vi "Test Save Animated GIF (Path).vi"(8 "error in (no error)":errorcluster) -> (0 "error out":errorcluster, 3 "Pass?":bool)   [LabVIEW 2020]
uses:
  G-Image/Image IO/Controls/Dither Type.ctl
  0f1b1910-5d7c-4507-bdef-12e0c9c3451f.vi
  G-Image/Image IO/Polymorphic VIs/Save Animated GIF Image (Path).vi
  G-Image/Image IO/Polymorphic VIs/Load Animated GIF Image (Path).vi
  G-Image/G-Image.lvlib
panel:
  out "Waveform Chart":cluster{dbl, dbl}(graph)={-0.06975647374412564, 0.4806308479691592}
  out "Array":cluster{string, "new picture":picture}[](array[cluster])
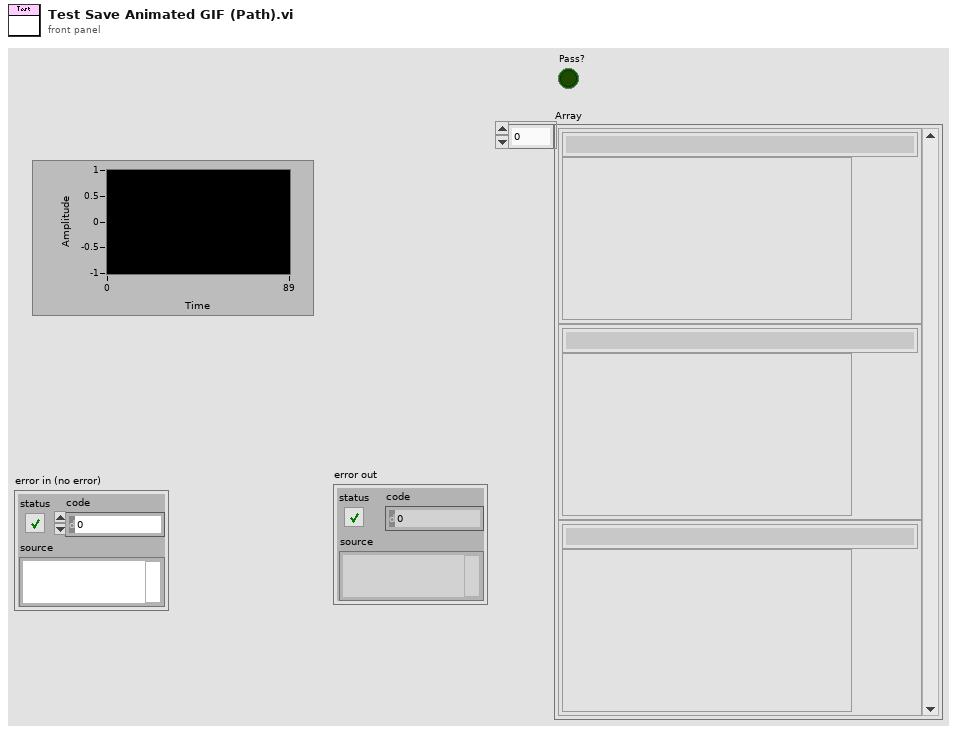
[diagram p1: front panel]
types:
  T1 = typedef "G-Image.lvlib/Dither Type.ctl" = enum32{"None", "Floyd-Steinberg"}
  T2 = typedef "imagedata.ctl" = cluster{"image type":i32, "image depth":i32, "image":u8[], "mask":u8[], "colors":u32[], "Rectangle":cluster{"left":i16, "top":i16, "right":i16, "bottom":i16}}
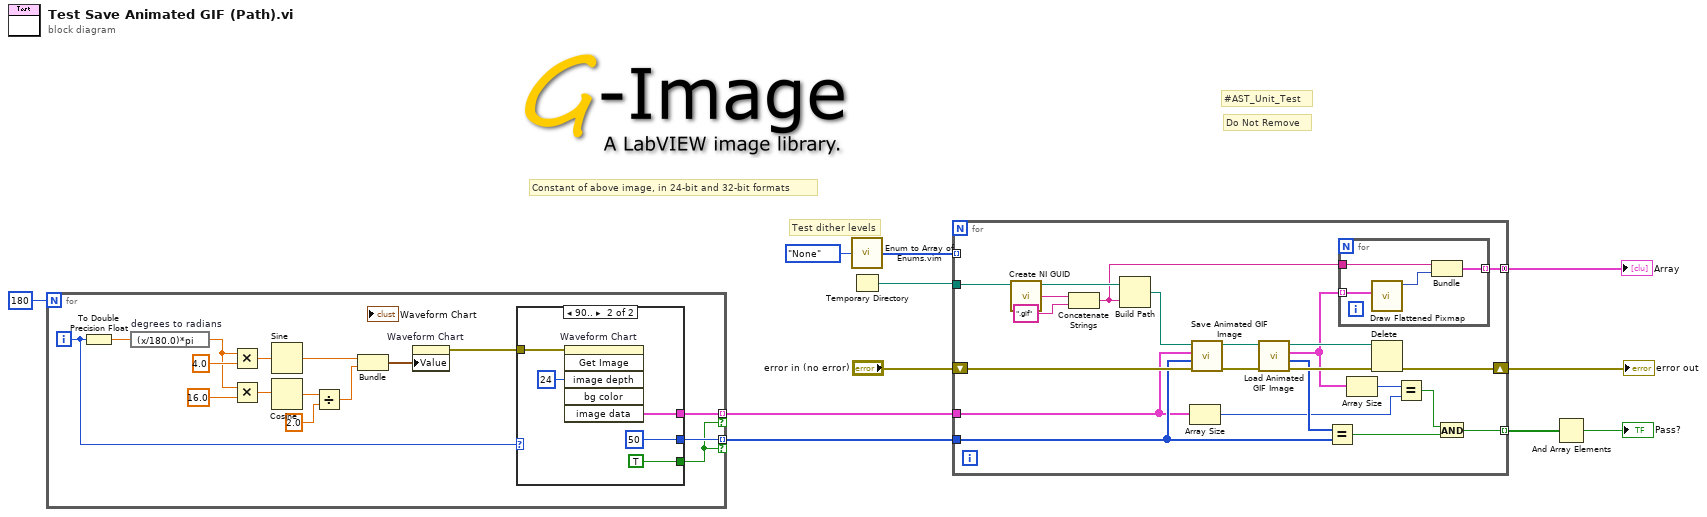
[diagram p0: block diagram]
diagram:
  # "Test dither levels"
  # "Constant of above image, in 24-bit and 32-bit formats"
  # "Do Not Remove"
  # "#AST_Unit_Test"
  n1 = for {
    N: 180 -> [_]
    tunnel: [w27] -> w4 mode=indexing if=w12
    tunnel: [w14] -> w3 mode=indexing if=w12
    i -> [w13]
    n2 = To Double Precision Float(number=w13) -> (double precision float=w24:dbl)
    n3 = expression code="(x/180.0)*pi" "degrees to radians"(w24) -> (w19:dbl)
    n4 = Multiply(x=w19, y=4.0) -> (x*y=w22:dbl)
    n5 = Multiply(x=w19, y=16.0) -> (x*y=w17:dbl)
    n6 = Sine(x=w22) -> (sin(x)=w21:dbl)
    n7 = Cosine(x=w17) -> (cos(x)=w20:dbl)
    n8 = Divide(x=w20, y=2.0) -> (x/y=w16:dbl)
    n9 = Bundle(w21, w16) -> (w23:cluster{dbl, dbl})  [unwired: 1 in]
    n10 = property on="Waveform Chart" class="WFChart (strict)"("Value"=w23) -> (error out=w26:errorcluster)  [unwired: 2 in, 1 out]
    n11 = case shown="90.." w13 {
      tunnel: [_ w31] -> w27
      tunnel: w26 -> [_ w30]
      tunnel: [_ 50] -> w14
      tunnel: [_ TRUE] -> w12
      frame Default {
      }
      frame 90.. {
        n12 = invoke on="Waveform Chart" class="WFChart (strict)" method="Get Image"(error in=w30, "image depth"=24 ("Image Depth")) -> ("image data"=w31:T2)  [unwired: 4 in, 5 out]
      }
    }
  }
  n13 = call "Enum to Array of Enums.vim"("enum"=Dither_Type."None" ("Dither (None)")) -> ("array of enums"=w6:T1[])
  n14 = Temporary Directory() -> (w10:path)
  n15 = for {
    tunnel: w10 -> [w50]
    shift-right: [w44] -> w8
    shift-left: "error in (no error)" -> [w53]
    tunnel: [w42] -> w9 mode=concatenating
    tunnel: w6 -> [_] mode=indexing
    tunnel: w4 -> [w39]
    tunnel: w3 -> [w40]
    tunnel: [w33] -> w2 mode=indexing
    n16 = call <vilib>:"Create NI GUID.vi"() -> ("NI GUID"=w51:string)
    n17 = Concatenate Strings(w51, ".gif" ("string")) -> (w43:string)
    n18 = Build Path(base path=w50, name or relative path=w43) -> (appended path=w49:path)
    n19 = Array Size(array=w39) -> (size(s)=w36:i32)
    n20 = call-poly "Save Animated GIF Image.vi"("error in (no error)"=w53, "Delays"=w40, "Frames"=w39, "Path In"=w49) -> ("error out"=w47:errorcluster, "Path Out"=w48:path)  [unwired: 6 in]
    n21 = call-poly "Load Animated GIF Image.vi"("error in (no error)"=w47, "Path In"=w48) -> ("error out"=w45:errorcluster, "Delays"=w41:i32[], "Frames"=w38:T2[], "Path Out"=w46:path)  [unwired: 6 in]
    n22 = Equal?(x=w41, y=w40) -> (x = y?=w34:bool)
    n23 = for {
      tunnel: w43 -> [w56]
      tunnel: [w55] -> w42 mode=indexing
      tunnel: w38 -> [w54] mode=indexing
      n24 = call <vilib>:"Draw Flattened Pixmap.vi"("image data"=w54) -> ("new picture"=w57:picture)  [unwired: 8 in]
      n25 = Bundle(w56, "new picture"=w57) -> (w55:cluster{string, "new picture":picture})  [unwired: 1 in]
    }
    n26 = Array Size(array=w38) -> (size(s)=w37:i32)
    n27 = Delete(path (use dialog)=w46, error in=w45) -> (error out=w44:errorcluster)  [unwired: 3 in, 2 out]
    n28 = Equal?(x=w37, y=w36) -> (x = y?=w35:bool)
    n29 = And(x=w35, y=w34) -> (x .and. y?=w33:bool)
  }
  "error out" <- w8
  "Array" <- w9
  n30 = And Array Elements(Boolean array=w2) -> (logical AND=→"Pass?":bool)
